vi "EventBuilder.constructor.vi"(0 "name":string, 2 "data in":string, 5 "error in (no error)":errorcluster) -> (14 "i ref out":refnum<vi>, 16 "data out":string, 19 "error out":errorcluster)   [LabVIEW 2014, in "EventBuilder.lvlib"]
doc: "constructor of THIS class\n\nLicense Agreement for this software:\n\nCopyright (C)\nGesellschaft für Schwerionenforschung, GSI\nPlanckstr. 1\n64291 Darmstadt\nGermany\n\nContact: D.Beck@gsi.de \n\nThis program is free software; you can redistribute it and/or modify it under the terms of the \nGNU General Public License as published by the Free Software Foundation; either version 2 of \nthe license, or (at your option) any later version.\n\nThis program is distributed in the hope that it will be useful, but WITHOUT ANY WARRANTY; \nwithout even the implied warranty of MERCHANTABILITY or FITNESS FOR A PARTICULAR PURPOSE. See the GNU General License for more details (http://www.gnu.org).\n\nGesellschaft für Schwerionenforschung, GSI\nPlanckstr. 1, 64291 Darmstadt, Germany\nFor all questions and ideas contact: M.Richter@gsi.de, H.Brand@gsi.de or D.Beck@gsi.de.\nLast update: 16-JUN-2004"
uses:
  EventBuilder.lvlib
  CSCore/BaseProcess/BaseProcess.lvlib
  CSCore/CSSystem/CSSystemLib/CSSystemLib.lvlib
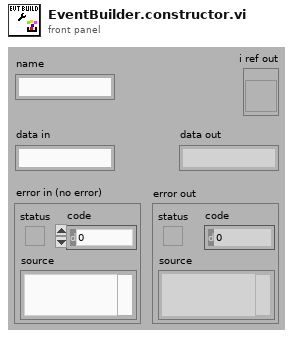
[diagram p1: front panel]
types:
  T1 = enum16{"SetAttribute", "GetAttribute", "CreateAttribute", "DestroyAttribute", "DestroyAllAtributes"}
  T2 = typedef "EventBuilder.lvlib/EventBuilder.i attribute.ctl" = cluster{"header":string, "DAQObjs":string[], "headerID":dbl, "eventID":i32, "dataDescriptionID":i32, "eventDataID":i32, "eventDataSize":i32, "dataDescriptionSize":i32}
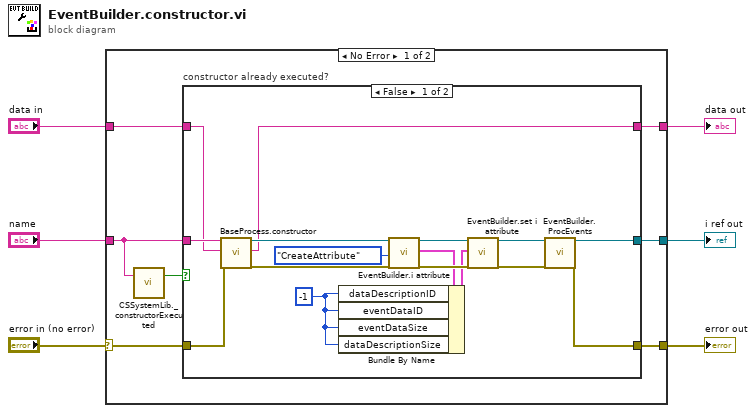
[diagram p0: block diagram]
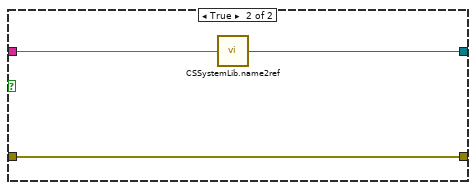
[diagram p2: hidden frame]
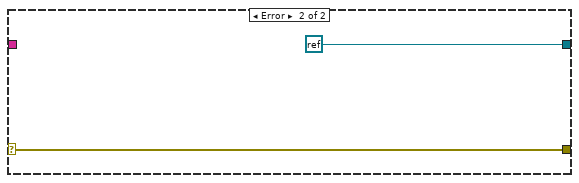
[diagram p3: hidden frame]
diagram:
  n1 = case shown="No Error" "error in (no error)" {
    selector: "error in (no error)" -> [w10 w33]
    tunnel: "name" -> [w8 _]
    tunnel: [w13 refnum<k0> refnum] -> w5
    tunnel: [w12 w33] -> w4
    tunnel: "data in" -> [w11 _]
    tunnel: [w7 _] -> w1
    frame No Error {
      n2 = call "CSSystemLib._constructorExecuted.vi"("name"=w8) -> ("constructor executed?"=w9:bool)  [unwired: 18 in]
      n3 = case "constructor already executed?" shown="False" w9 {
        tunnel: w8 -> [w26 w32]
        tunnel: [w23 w31] -> w13
        tunnel: [w22 w30] -> w12
        tunnel: w11 -> [w25 _]
        tunnel: w10 -> [w24 w30]
        tunnel: [w14 _] -> w7
        frame False {
          w15 = -1 ("dataDescriptionID")
          n4 = call "BaseProcess.constructor.vi"("name"=w26, "data in"=w25, "error in (no error)"=w24) -> ("i ref out"=w29:refnum<vi>, "data out"=w14:string, "error out"=w28:errorcluster)  [unwired: 14 in]
          n5 = call "EventBuilder.i attribute.vi"("VI Refnum"=w29, "Action"=T1."CreateAttribute", "error in (no error)"=w28) -> ("VI Refnum out"=w21:refnum<vi>, "CLASS.i attribute out"=w19:T2, "error out"=w20:errorcluster)  [unwired: 14 in]
          n6 = Bundle By Name(cluster=w19, "dataDescriptionID"=w15, "eventDataID"=w15, "eventDataSize"=w15, "dataDescriptionSize"=w15) -> (w18:T2)
          n7 = call "EventBuilder.set i attribute.vi"("i ref in"=w21, "i attribute"=w18, "error in (no error)"=w20) -> ("i ref out"=w17:refnum<vi>, "error out"=w16:errorcluster)  [unwired: 15 in]
          n8 = call "EventBuilder.ProcEvents.vi"("i ref in"=w17, "error in (no error)"=w16) -> ("i ref out"=w23:refnum<vi>, "error out"=w22:errorcluster)  [unwired: 16 in]
        }
        frame True {
          n9 = call "CSSystemLib.name2ref.vi"("name"=w32) -> ("obj refnum"=w31:refnum<vi>)
        }
      }
    }
    frame Error {
    }
  }
  "i ref out" <- w5
  "error out" <- w4
  "data out" <- w1
